vi "Status.vi"() -> ()   [LabVIEW 2016]
panel:
  out "Status":T1
  # "Region 3"
  # "Region 2"
  # "Region 1"
  # "Position 2"
  # "Position 1"
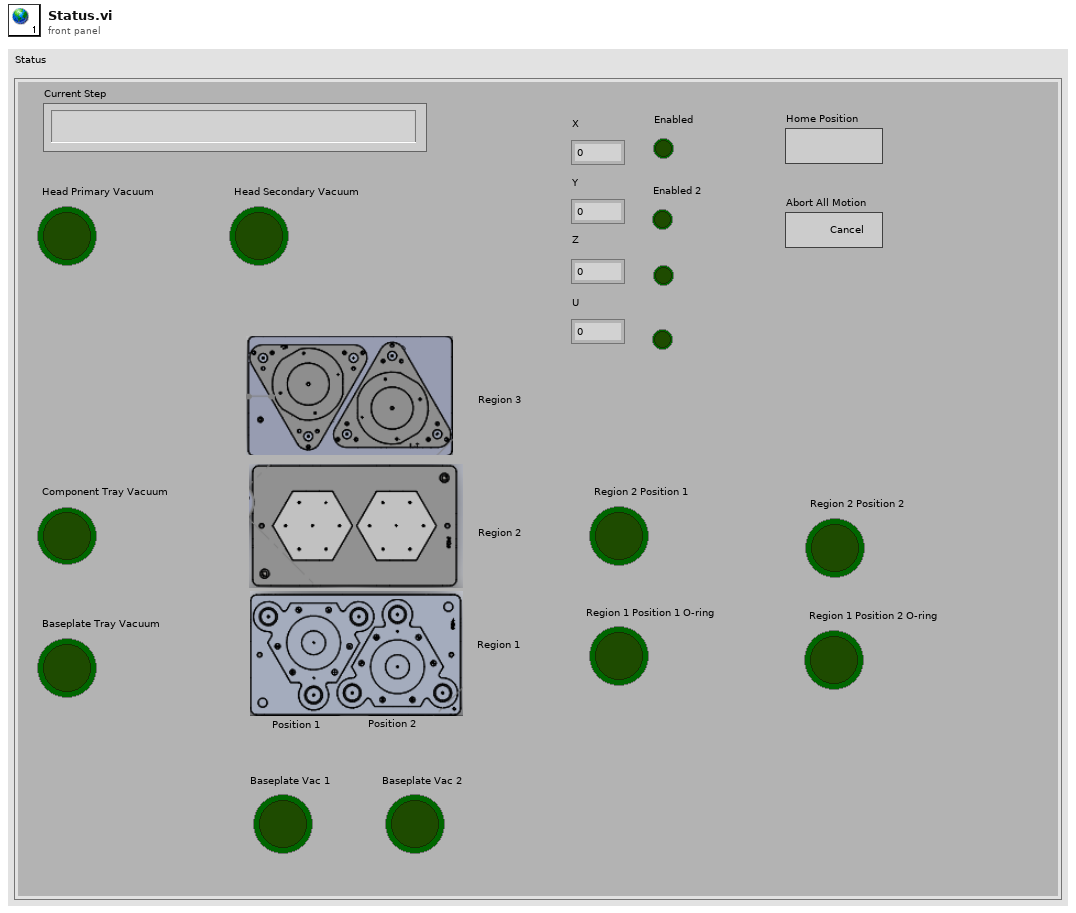
[diagram p1: front panel]
types:
  T1 = cluster{"Current Step":string, "Baseplate Tray Vacuum":bool, "Component Tray Vacuum":bool, "Head Primary Vacuum":bool, "Head Secondary Vacuum":bool, "Region 1 Position 1 O-ring":bool, "Region 1 Position 2 O-ring":bool, "Region 2 Position 1":bool, "Region 2 Position 2":bool, "X":dbl, "Y":dbl, "Z":dbl, "U":dbl, "Home Position":bool, "Enabled":bool, "Enabled 2":bool, bool, bool, "Abort All Motion":bool, "Baseplate Vac 1":bool, "Baseplate Vac 2":bool}
diagram:
